vi "MED_AMPL.vi"(11 "Boolean":bool) -> ()   [LabVIEW 2009]
panel:
  in  "Directorio scripts matlab":path=path "C:/Users/franjas/Documents/rutinas-calibracion-slm"
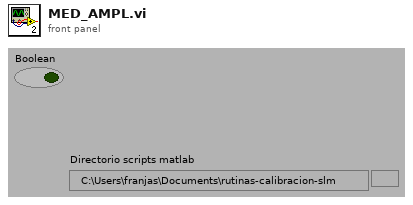
[diagram p1: front panel]
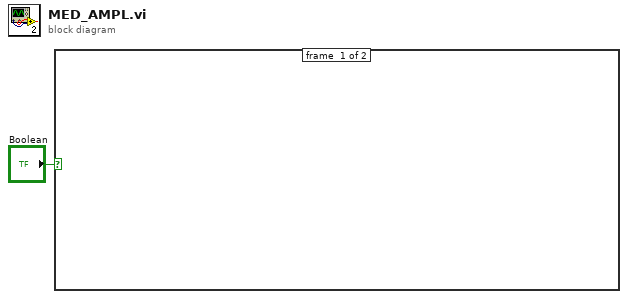
[diagram p0: block diagram]
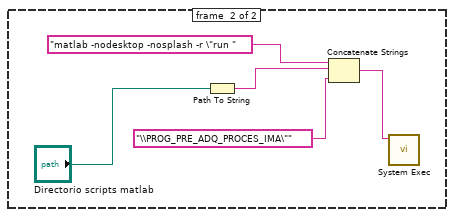
[diagram p2: hidden frame]
diagram:
  n1 = case shown="True" "Boolean" {
    frame #0 {
    }
    frame #1 {
      n2 = Path To String(path="Directorio scripts matlab") -> (string=w2:string)
      n3 = Concatenate Strings("matlab -nodesktop -nosplash -r \"run " ("command line"), w2, "\\PROG_PRE_ADQ_PROCES_IMA\"" ("command line")) -> (w4:string)
      n4 = call <vilib>:"System Exec.vi"("command line"=w4) -> ()  [unwired: 7 in, 4 out]
    }
  }
